vi "ReportGenerator.Title.vi"(8 "error in (no error)":errorcluster, 9 "Font":T1, 10 "Title":string, 11 "NI_report in":refnum<class "NI_report.lvclass">) -> (0 "error out":errorcluster, 3 "NI_report out":refnum<class "NI_report.lvclass">)   [LabVIEW 2019, in "Tools.lvlib"]
uses:
  <vilib>/Utility/NIReport.llb/NI_report.lvclass
  <vilib>/Utility/NIReport.llb/Append Report Text (str wrap).vi
  Tools.lvlib
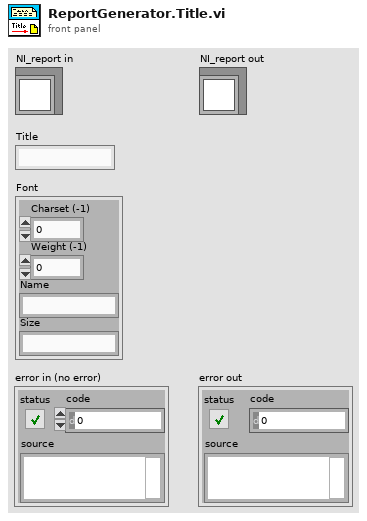
[diagram p1: front panel]
types:
  T1 = cluster{"Charset (-1)":i16, "Weight (-1)":i16, "Name":string, "Size":string}
  T2 = cluster{"Italic":enum16{"Italic Unchanged", "Italic On", "Italic Off"}, "Strike Through":enum16{"Strike Through Unchanged", "Strike Through On", "Strike Through Off"}, "Underline":enum16{"Underline Unchanged", "Underline On", "Underline Off"}, "Bold":enum16{"Bold Unchanged", "Bold On", "Bold Off"}}
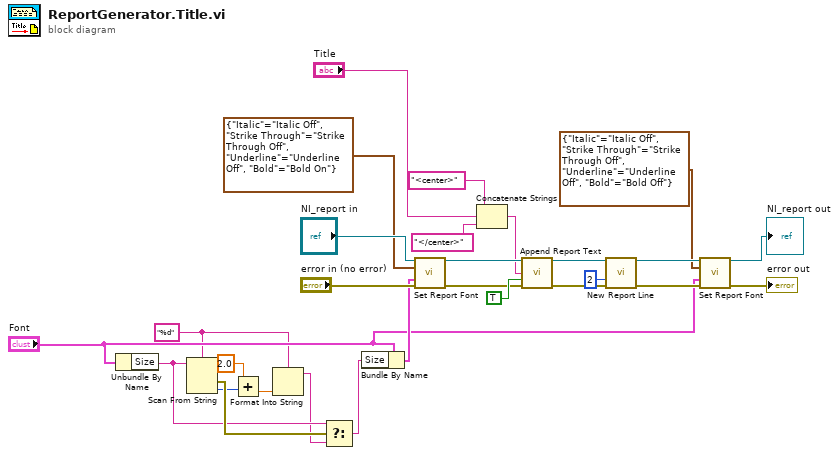
[diagram p0: block diagram]
diagram:
  w4 = "%d" ("format string")
  n1 = Unbundle By Name("Font") -> ("Size"=w18:string)
  n2 = Scan From String(format string=w4, input string=w18) -> (error out=w19:errorcluster, output 1=w3:i32)  [unwired: 3 in, 2 out]
  n3 = Add(x=2.0, y=w3) -> (x+y=w2:dbl)
  n4 = Format Into String(format string=w4, w2) -> (resulting string=w17:string)  [unwired: 2 in, 1 out]
  n5 = Select(t=w18, s=w19, f=w17) -> (s? t:f=w5:string)
  n6 = Bundle By Name(cluster="Font", "Size"=w5) -> (w11:T1)
  n7 = call-dynamic "Set Report Font.vi"("report in"="NI_report in", "text options"=T2 {"Italic"=enum."Italic Off", "Strike Through"=enum."Strike Through Off", "Underline"=enum."Underline Off", "Bold"=enum."Bold On"}, "font settings"=w11, "error in (no error)"="error in (no error)") -> ("report out"=w20:refnum<class "NI_report.lvclass">, "error out"=w21:errorcluster)  [unwired: 9 in, 1 out]
  n8 = Concatenate Strings("<center>" ("string"), "Title", "</center>" ("string")) -> (w9:string)
  n9 = call-poly <vilib>:"Append Report Text.vi"("report in"=w20, "text"=w9, "append on new line? (F)"=TRUE, "error in (no error)"=w21) -> ("report out"=w16:refnum<class "NI_report.lvclass">, "error out"=w15:errorcluster)  [unwired: 8 in, 2 out]
  n10 = call-dynamic "New Report Line.vi"("report in"=w16, "number of lines (1)"=2, "error in (no error)"=w15) -> ("report out"=w13:refnum<class "NI_report.lvclass">, "error out"=w14:errorcluster)  [unwired: 11 in]
  n11 = call-dynamic "Set Report Font.vi"("report in"=w13, "text options"=T2 {"Italic"=enum."Italic Off", "Strike Through"=enum."Strike Through Off", "Underline"=enum."Underline Off", "Bold"=enum."Bold Off"}, "font settings"="Font", "error in (no error)"=w14) -> ("report out"=→"NI_report out":refnum<class "NI_report.lvclass">, "error out"=→"error out":errorcluster)  [unwired: 9 in, 1 out]
